vi "WaitOnProcessSync.vi"(8 "error in (no error)":errorcluster, 9 "timeout in ms (-1)":i32=-1, 11 "SMO":refnum<class "SMO.lvclass">) -> (0 "error out":errorcluster, 1 "Don't run?":bool, 3 "SMO out":refnum<class "SMO.lvclass">)   [LabVIEW 2019, in "SMO.lvclass"]
doc: "This method is used to synchronize processes during launch and shutdown\n\nNote: This method is overridable by descendant\n\n---------------------------------------------------------------\nJKI State Machine Objects™\nhttp://jki.net/state-machine-objects/\nCopyright (C) 2005-2015, JKI <info@jki.net>\nALL RIGHTS RESERVEDJKI State Machine Objects (SMO) 1.3.0.56\nJKI - JKI\nCopyright (c) 2017, JKI"
uses:
  SMO.lvclass
panel:
  # "For instructions on how to use the JKI State Machine Objects, examples and video tutorials, visit:\nhttp://jki.net/state-machine-objects/\n\nJKI State Machine Objects™\nhttp://jki.net/state-machine-objects/\nCopyright (C) 2005-2015, JKI <info@jki.net>\nALL RIGHTS RESERVED"
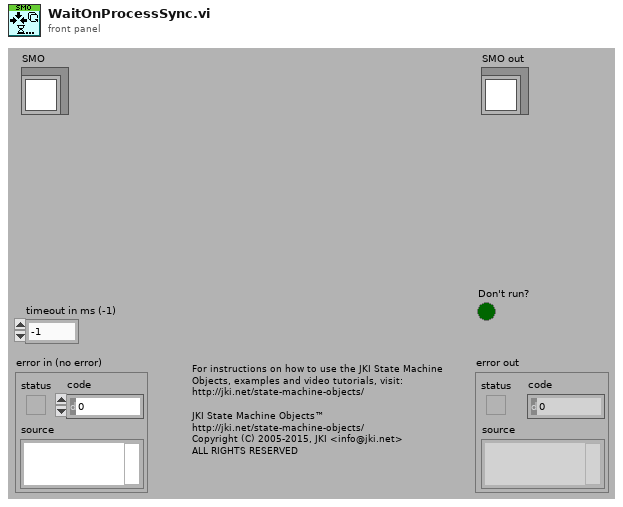
[diagram p1: front panel]
types:
  T1 = typedef "SMO.lvclass/SMOState --Enum.ctl" = enum16{"unknown", "Created", "Started", "Stopped"}
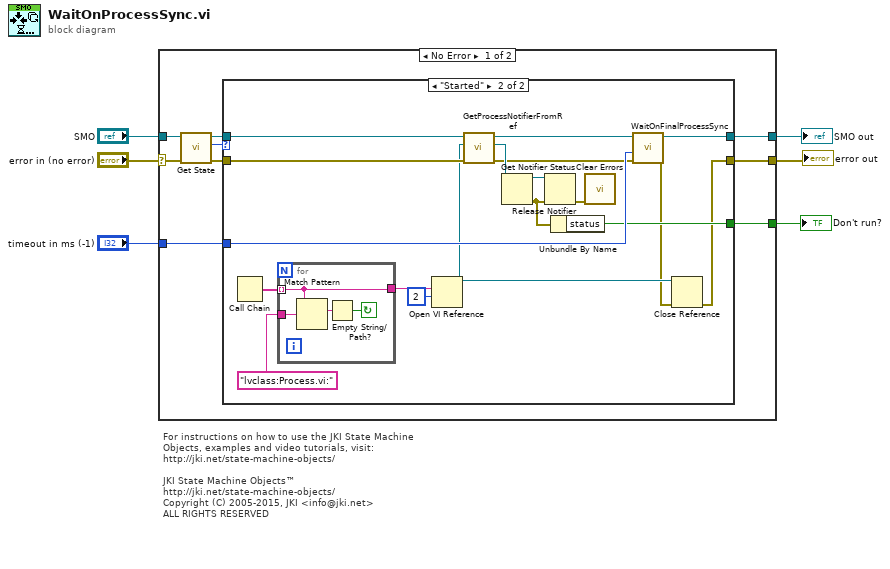
[diagram p0: block diagram]
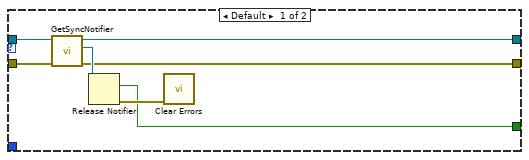
[diagram p2: hidden frame]
diagram:
  # "For instructions on how to use the JKI State Machine Objects, examples and video tutorials, visit:\nhttp://jki.net/state-machine-objects/\n\nJKI State Machine Objects™\nhttp://jki.net/state-machine-objects/\nCopyright (C) 2005-2015, JKI <info@jki.net>\nALL RIGHTS RESERVED"
  n1 = case shown="No Error" "error in (no error)" {
    selector: "error in (no error)" -> [w14 w46]
    tunnel: [w12 w46] -> w5
    tunnel: [w13 w45] -> w4
    tunnel: "SMO" -> [w15 w45]
    tunnel: "timeout in ms (-1)" -> [w11 _]
    tunnel: [w7 _] -> w1
    frame No Error {
      n2 = call "Get State.vi"("error in (no error)"=w14, "SMO"=w15) -> ("error out"=w9:errorcluster, "SMO State"=w8:T1, "SMO out"=w10:refnum<class "SMO.lvclass">)  [unwired: 7 in]
      n3 = case shown="\"Started\"" w8 {
        tunnel: [w18 w39] -> w13
        tunnel: [w20 w26] -> w12
        tunnel: w10 -> [w19 w35]
        tunnel: w9 -> [w21 w33]
        tunnel: w11 -> [_ w40]
        tunnel: [w16 w30] -> w7
        frame Default {
          n4 = call "GetSyncNotifier.vi"("error in (no error)"=w21, "SMO in"=w19) -> ("error out"=w20:errorcluster, "Sync Notifier"=w22:refnum<notifier>, "SMO out"=w18:refnum<class "SMO.lvclass">)  [unwired: 7 in]
          n5 = Release Notifier(notifier=w22) -> (last notification=w16:bool, error out=w17:errorcluster)  [unwired: 2 in, 1 out]
          n6 = call <vilib>:"Clear Errors.vi"("error in (no error)"=w17) -> ()  [unwired: 5 in, 2 out]
        }
        frame "Started" {
          n7 = Call Chain() -> (call chain=w25:string[])
          n8 = for {
            tunnel: w25 -> [w41] mode=indexing
            tunnel: "lvclass:Process.vi:" -> [w44]
            tunnel: [w41] -> w24
            stop <- w42 continue-if-true
            n9 = Match Pattern(string=w41, regular expression=w44) -> (match substring=w43:string)  [unwired: 1 in, 3 out]
            n10 = Empty String/Path?(string/path=w43) -> (empty?=w42:bool)
          }
          n11 = Open VI Reference(vi path=w24, options=2) -> (vi reference=w28:refnum<vi>)  [unwired: 4 in, 1 out]
          n12 = call "GetProcessNotifierFromRef.vi"("error in (no error)"=w33, "Process VI Refnum"=w28, "SMO"=w35) -> ("error out"=w32:errorcluster, "Sync Notifier"=w36:refnum<notifier>, "SMO out"=w34:refnum<class "SMO.lvclass">)  [unwired: 6 in]
          n13 = Get Notifier Status(notifier=w36) -> (notifier out=w38:refnum<notifier>, error out=w31:errorcluster)  [unwired: 1 in, 3 out]
          n14 = Release Notifier(notifier=w38, error in (no error)=w31) -> (error out=w29:errorcluster)  [unwired: 1 in, 2 out]
          n15 = Unbundle By Name(w31) -> ("status"=w30:bool)
          n16 = call <vilib>:"Clear Errors.vi"("error in (no error)"=w29) -> ()  [unwired: 5 in, 2 out]
          n17 = call "WaitOnFinalProcessSync.vi"("error in (no error)"=w32, "timeout in ms (-1)"=w40, "SMO"=w34) -> ("error out"=w27:errorcluster, "SMO out"=w39:refnum<class "SMO.lvclass">)  [unwired: 7 in]
          n18 = Close Reference(reference=w28, error in (no error)=w27) -> (error out=w26:errorcluster)
        }
      }
    }
    frame Error {
    }
  }
  "error out" <- w5
  "SMO out" <- w4
  "Don't run?" <- w1
